vi "Write Acquisition Config.vi"(6 "Image Name":string, 7 "Image Path":string, 8 "error in (no error)":errorcluster, 9 "# Exposure":dbl, 10 "Exposure Time":dbl, 11 "CCDCamera in":refnum<class "CCDCamera.lvclass">) -> (0 "error out":errorcluster, 3 "CCDCamera out":refnum<class "CCDCamera.lvclass">)   [LabVIEW 2018, in "CCDCamera.lvclass"]
doc: "This VI writes the exposure time, the number of exposures, the image path, and the image name to the class."
uses:
  CCDCamera.lvclass
  CCDCamera.lvclass/CCDCamera.ctl
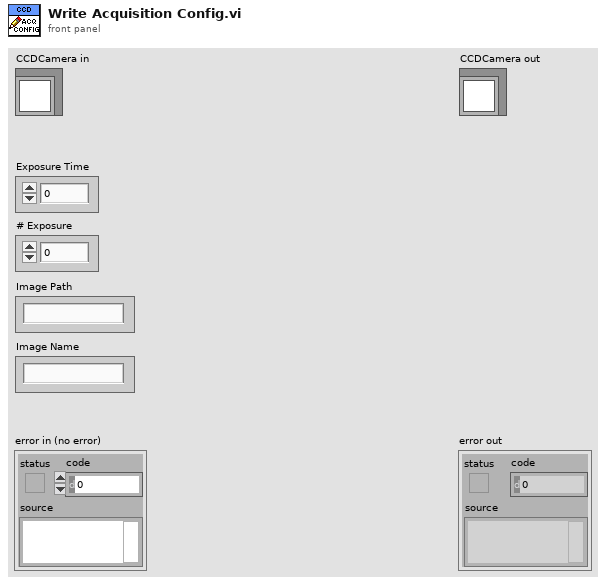
[diagram p1: front panel]
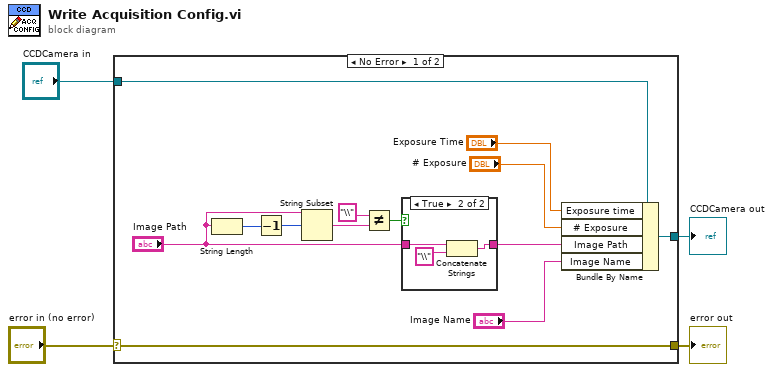
[diagram p0: block diagram]
diagram:
  n1 = case shown="No Error" "error in (no error)" {
    selector: "error in (no error)" -> [w17 w23]
    tunnel: [w17 w23] -> w3
    tunnel: [w15 w22] -> w1
    tunnel: "CCDCamera in" -> [w16 w22]
    frame No Error {
      n2 = String Length(string="Image Path") -> (length=w6:i32)
      n3 = Decrement(x=w6) -> (x-1=w5:i32)
      n4 = String Subset(string="Image Path", offset (0)=w5) -> (substring=w9:string)  [unwired: 1 in]
      n5 = Not Equal?(x="\\", y=w9) -> (x != y?=w11:bool)
      n6 = case shown="True" w11 {
        tunnel: "Image Path" -> [w18 w20]
        tunnel: [w18 w19] -> w8
        frame False {
        }
        frame True {
          n7 = Concatenate Strings(w20, "\\" ("x")) -> (w19:string)
        }
      }
      n8 = Bundle By Name(cluster=w16, "Exposure time"="Exposure Time", "# Exposure"="# Exposure", "Image Path"=w8, "Image Name"="Image Name") -> (w15:refnum<class "CCDCamera.lvclass">)
    }
    frame Error {
    }
  }
  "error out" <- w3
  "CCDCamera out" <- w1
